vi "Test Case, MD5 Buffer.vi"() -> ()   [LabVIEW 2010]
panel:
  out "Buffer MD5 message-digest (CRM)":string
  out "File MD5 message-digest (NI)":string
  out "match?":bool
  in  "filepath":path=path "C:/Documents and Settings/user/Desktop/Claytons Archive/Calculate Statistics.vi"
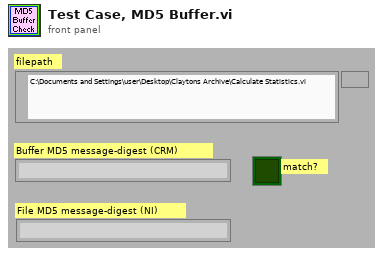
[diagram p1: front panel]
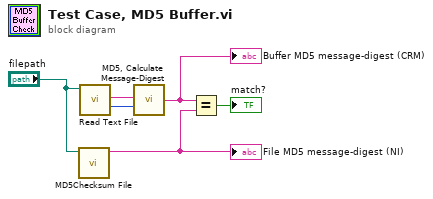
[diagram p0: block diagram]
diagram:
  n1 = call <vilib>:"MD5Checksum File.vi"("Path"="filepath") -> ("MD5 message-digest"=w3:string)  [unwired: 9 in, 1 out]
  "File MD5 message-digest (NI)" <- w3
  n2 = call "Read Text File.vi"("filepath"="filepath") -> ("size (bytes)"=w5:i64, "data"=w6:string)  [unwired: 8 in, 1 out]
  n3 = call "MD5, Calculate Message-Digest.vi"("size (in bytes)"=w5, "data"=w6) -> ("MD5 message-digest"=w1:string)  [unwired: 2 in]
  "Buffer MD5 message-digest (CRM)" <- w1
  n4 = Equal?(x=w1, y=w3) -> (x = y?=→"match?":bool)
